vi "Format Status String.vi"(10 "initial string":string, 11 "format string":string) -> (2 "initial string out":string, 3 "format string out":string)   [LabVIEW 2019, in "Instrument.Lockin.lvclass"]
uses:
  Instrument.Lockin.lvclass
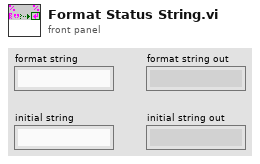
[diagram p1: front panel]
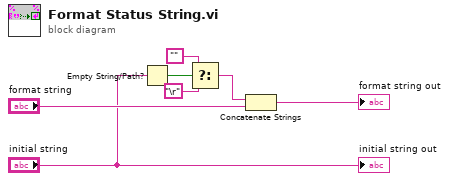
[diagram p0: block diagram]
diagram:
  n1 = Empty String/Path?(string/path="initial string") -> (empty?=w2:bool)
  n2 = Select(t="", s=w2, f="\r") -> (s? t:f=w4:string)
  n3 = Concatenate Strings(w4, "format string") -> (→"format string out":string)
  "initial string out" <- "initial string"
